vi "RT Variables Init.vi"(8 "error in (no error)":errorcluster) -> (0 "error out":errorcluster, 3 "Time has Elapsed?":bool)   [LabVIEW 2017]
doc: "Setup default values to all used network-published\nshared variables and wait for their application"
uses:
  RT Status.ctl
  RT Loop Status.ctl
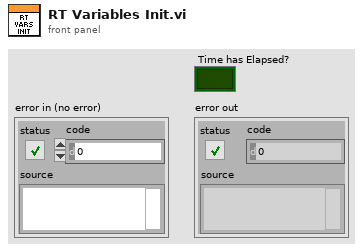
[diagram p1: front panel]
types:
  T1 = typedef "RT Status.ctl" = cluster{"Status TCL1":T2, "Status TCL2":T2, "Status NPL":T2, "Connected?":bool}
  T2 = typedef "RT Loop Status.ctl" = cluster{"Duration, us":dbl, "Late Counter":i32, "Timeout, us":u32}
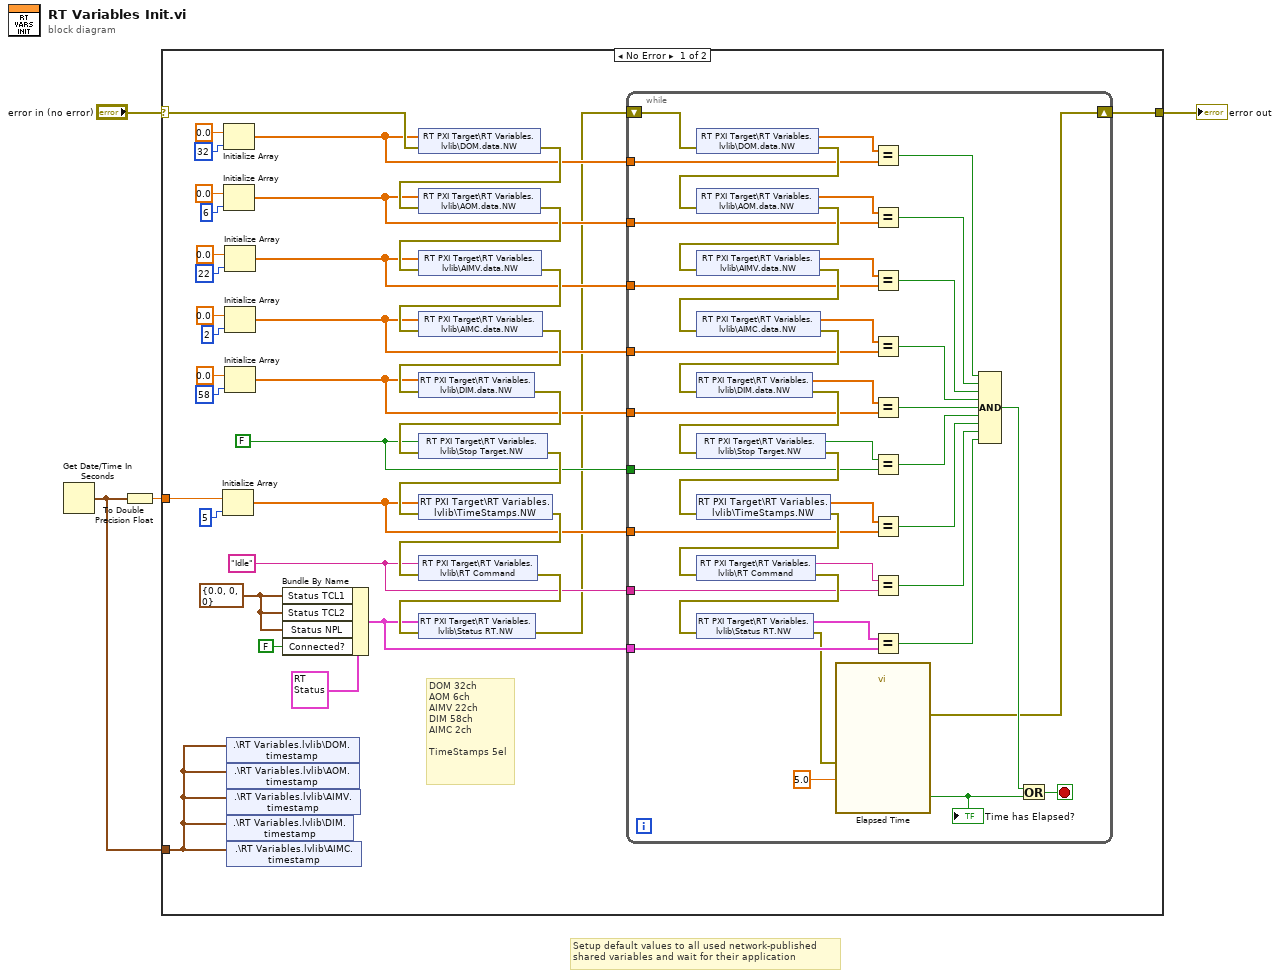
[diagram p0: block diagram]
diagram:
  # "Setup default values to all used network-published\nshared variables and wait for their application"
  n1 = Get Date/Time In Seconds() -> (seconds since 1Jan1904=w1:timestamp)
  n2 = To Double Precision Float(number=w1) -> (double precision float=w2:dbl)
  n3 = case shown="No Error" "error in (no error)" {
    selector: "error in (no error)" -> [w17 w83]
    tunnel: [w7 w83] -> w3
    tunnel: w2 -> [w29 _]
    tunnel: w1 -> [w5 _]
    frame No Error {
      w27 = T2 {"Duration, us"=0.0, "Late Counter"=0, "Timeout, us"=0} ("Status TCL1")
      w9 = "Idle" ("RT Command")
      w11 = FALSE ("Stop Target.NW")
      # "DOM 32ch\nAOM 6ch\nAIMV 22ch\nDIM 58ch\nAIMC 2ch\n\nTimeStamps 5el"
      n4 = Initialize Array(w29, 5 ("dimension size")) -> (w10:dbl[])
      n5 = Initialize Array(0.0 ("element"), 32 ("dimension size")) -> (w16:dbl[])
      n6 = Initialize Array(0.0 ("element"), 6 ("dimension size")) -> (w15:dbl[])
      n7 = Initialize Array(0.0 ("element"), 22 ("dimension size")) -> (w14:dbl[])
      n8 = Initialize Array(0.0 ("element"), 2 ("dimension size")) -> (w13:dbl[])
      n9 = Initialize Array(0.0 ("element"), 58 ("dimension size")) -> (w12:dbl[])
      n10 = shared-variable ".\\RT Variables.lvlib\\DOM.timestamp"(w5) -> ()  [unwired: 1 in, 1 out]
      n11 = shared-variable ".\\RT Variables.lvlib\\AOM.timestamp"(w5) -> ()  [unwired: 1 in, 1 out]
      n12 = shared-variable ".\\RT Variables.lvlib\\AIMV.timestamp"(w5) -> ()  [unwired: 1 in, 1 out]
      n13 = shared-variable ".\\RT Variables.lvlib\\DIM.timestamp"(w5) -> ()  [unwired: 1 in, 1 out]
      n14 = shared-variable ".\\RT Variables.lvlib\\AIMC.timestamp"(w5) -> ()  [unwired: 1 in, 1 out]
      n15 = Bundle By Name(cluster=T1 {"Status TCL1"={"Duration, us"=0.0, "Late Counter"=0, "Timeout, us"=0}, "Status TCL2"={"Duration, us"=0.0, "Late Counter"=0, "Timeout, us"=0}, "Status NPL"={"Duration, us"=0.0, "Late Counter"=0, "Timeout, us"=0}, "Connected?"=FALSE} ("RT Status"), "Status TCL1"=w27, "Status TCL2"=w27, "Status NPL"=w27, "Connected?"=FALSE) -> (w8:T1)
      n16 = shared-variable "RT PXI Target\\RT Variables.lvlib\\DOM.data.NW"(w16, error in=w17) -> (error out=w25:errorcluster)
      n17 = shared-variable "RT PXI Target\\RT Variables.lvlib\\AOM.data.NW"(w15, error in=w25) -> (error out=w24:errorcluster)
      n18 = shared-variable "RT PXI Target\\RT Variables.lvlib\\AIMV.data.NW"(w14, error in=w24) -> (error out=w23:errorcluster)
      n19 = shared-variable "RT PXI Target\\RT Variables.lvlib\\AIMC.data.NW"(w13, error in=w23) -> (error out=w22:errorcluster)
      n20 = shared-variable "RT PXI Target\\RT Variables.lvlib\\DIM.data.NW"(w12, error in=w22) -> (error out=w21:errorcluster)
      n21 = shared-variable "RT PXI Target\\RT Variables.lvlib\\Stop Target.NW"(w11, error in=w21) -> (error out=w20:errorcluster)
      n22 = shared-variable "RT PXI Target\\RT Variables.lvlib\\TimeStamps.NW"(w10, error in=w20) -> (error out=w19:errorcluster)
      n23 = shared-variable "RT PXI Target\\RT Variables.lvlib\\RT Command"(w9, error in=w19) -> (error out=w18:errorcluster)
      n24 = shared-variable "RT PXI Target\\RT Variables.lvlib\\Status RT.NW"(w8, error in=w18) -> (error out=w6:errorcluster)
      n25 = while {
        shift-right: [w41] -> w7
        shift-left: w6 -> [w82]
        tunnel: w16 -> [w73]
        tunnel: w15 -> [w72]
        tunnel: w14 -> [w71]
        tunnel: w13 -> [w70]
        tunnel: w12 -> [w69]
        tunnel: w11 -> [w68]
        tunnel: w10 -> [w67]
        tunnel: w9 -> [w66]
        tunnel: w8 -> [w65]
        stop <- w42 stop-if-true
        n26 = shared-variable "RT PXI Target\\RT Variables.lvlib\\DOM.data.NW"(error in=w82) -> (w61:dbl[], error out=w81:errorcluster)
        n27 = shared-variable "RT PXI Target\\RT Variables.lvlib\\AOM.data.NW"(error in=w81) -> (w64:dbl[], error out=w80:errorcluster)
        n28 = shared-variable "RT PXI Target\\RT Variables.lvlib\\AIMV.data.NW"(error in=w80) -> (w63:dbl[], error out=w79:errorcluster)
        n29 = shared-variable "RT PXI Target\\RT Variables.lvlib\\AIMC.data.NW"(error in=w79) -> (w62:dbl[], error out=w78:errorcluster)
        n30 = shared-variable "RT PXI Target\\RT Variables.lvlib\\DIM.data.NW"(error in=w78) -> (w60:dbl[], error out=w77:errorcluster)
        n31 = shared-variable "RT PXI Target\\RT Variables.lvlib\\Stop Target.NW"(error in=w77) -> (w59:bool, error out=w76:errorcluster)
        n32 = shared-variable "RT PXI Target\\RT Variables.lvlib\\TimeStamps.NW"(error in=w76) -> (w58:dbl[], error out=w75:errorcluster)
        n33 = shared-variable "RT PXI Target\\RT Variables.lvlib\\RT Command"(error in=w75) -> (w57:string, error out=w74:errorcluster)
        n34 = shared-variable "RT PXI Target\\RT Variables.lvlib\\Status RT.NW"(error in=w74) -> (w56:T1, error out=w55:errorcluster)
        n35 = call "Elapsed Time"("Time Target (s)"=5.0, "error in (no error)"=w55) -> ("Time has Elapsed"=w44:bool, "error out"=w41:errorcluster)  [unwired: 10 in, 6 out]
        "Time has Elapsed?" <- w44
        n36 = Equal?(x=w61, y=w73) -> (x = y?=w53:bool)
        n37 = Equal?(x=w64, y=w72) -> (x = y?=w52:bool)
        n38 = Equal?(x=w63, y=w71) -> (x = y?=w51:bool)
        n39 = Equal?(x=w62, y=w70) -> (x = y?=w50:bool)
        n40 = Equal?(x=w60, y=w69) -> (x = y?=w49:bool)
        n41 = Equal?(x=w59, y=w68) -> (x = y?=w48:bool)
        n42 = Equal?(x=w58, y=w67) -> (x = y?=w47:bool)
        n43 = Equal?(x=w57, y=w66) -> (x = y?=w46:bool)
        n44 = Equal?(x=w56, y=w65) -> (x = y?=w45:bool)
        n45 = Compound Arithmetic op=AND(w53, w52, w51, w50, w49, w48, w47, w46, w45) -> (w43:bool)
        n46 = Or(x=w43, y=w44) -> (x .or. y?=w42:bool)
      }
    }
    frame Error {
    }
  }
  "error out" <- w3
